vi "Modbus RT Driver - Display configuration Details.vi"(9 "Array 2":T1[](array[typedef]), 11 "Array":T3[](array[typedef])) -> ()   [LabVIEW 2014, in "Modbus Engine.lvlib"]
uses:
  Modbus Engine.lvlib
  XML Deserializer/XML VIs/API/Controls/Modbus_Items.ctl
  XML Deserializer/XML VIs/API/Controls/Modbus_Item_Type.ctl
  Shared/FIFO Indexes.ctl
  <vilib>/NI Veristand/Custom Device API/Custom Device Channel Type.ctl
  <vilib>/NI Veristand/Custom Device Tools/Custom Device Utility Library/Custom Device Utility Library.lvlib
  Shared/Modbus Shared.lvlib
  <vilib>/NI Veristand/Custom Device API/Custom Device API.lvlib
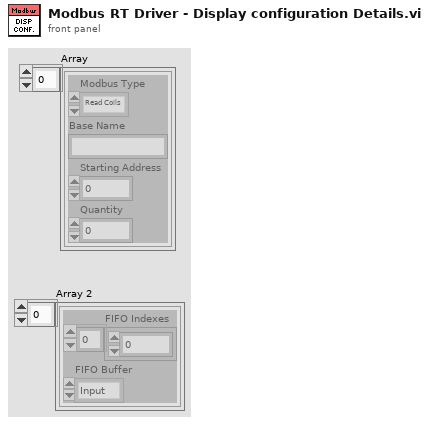
[diagram p1: front panel]
types:
  T1 = typedef "Modbus Shared.lvlib/FIFO Indexes.ctl" = cluster{"FIFO Indexes":i32[], "FIFO Buffer":T2}
  T2 = typedef "Custom Device API.lvlib/Custom Device Channel Type.ctl" = enum16{"Input", "Output"}
  T3 = typedef "Modbus Shared.lvlib/Modbus_Items.ctl" = cluster{"Modbus Type":T4, "Base Name":string, "Starting Address":u16, "Quantity":u16}
  T4 = typedef "Modbus Shared.lvlib/Modbus_Item_Type.ctl" = enum16{"Read Coils", "Read Discrete Inputs", "Read Holding Registers", "Read Input Registers", "Write Multiple Coils", "Write Multiple Holding Registers", "Write Single Coil", "Write Single Holding Register", "Write Multiple Discrete Inputs", "Write Multiple Input Registers"}
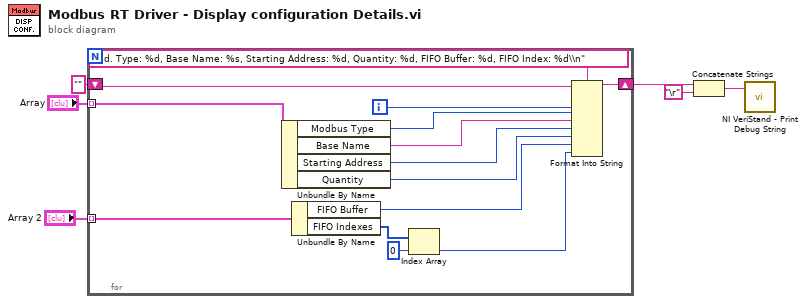
[diagram p0: block diagram]
diagram:
  n1 = for {
    tunnel: "Array" -> [w18] mode=indexing
    shift-right: [w20] -> w5
    shift-left: "" -> [w19]
    tunnel: "Array 2" -> [w11] mode=indexing
    i -> [w16]
    n2 = Unbundle By Name(w18) -> ("Modbus Type"=w15:T4, "Base Name"=w14:string, "Starting Address"=w13:u16, "Quantity"=w12:u16)
    n3 = Unbundle By Name(w11) -> ("FIFO Buffer"=w8:T2, "FIFO Indexes"=w10:i32[])
    n4 = Index Array(array=w10, index=0) -> (element=w7:i32)
    n5 = Format Into String(format string="%d. Type: %d, Base Name: %s, Starting Address: %d, Quantity: %d, FIFO Buffer: %d, FIFO Index: %d\\n", initial string=w19, w16, w15, w14, w13, w12, w8, w7) -> (resulting string=w20:string)  [unwired: 1 in, 1 out]
  }
  n6 = Concatenate Strings(w5, "\r") -> (w4:string)
  n7 = call <vilib>:"NI VeriStand - Print Debug String.vi"("Message"=w4) -> ()  [unwired: 10 in, 1 out]
